vi "Init with Value.vi"(8 "error in":errorcluster, 10 "Value":variant, 11 "Check Box in":refnum<class "Check Box.lvclass">) -> (0 "error out":errorcluster, 3 "Check Box out":refnum<class "Check Box.lvclass">)   [LabVIEW 2024, in "SourceGrid.lvlib" / "Check Box.lvclass"]
uses:
  Check Box.lvclass
  Check Box.lvclass/Check Box.ctl
  Cells/Cell/Cell.lvclass
  D:/git/Sourcegrid-LabVIEW/source/Cells/Cell/Cell.lvclass
  D:/git/Sourcegrid-LabVIEW/source/Editors/Check Box/Check Box.lvclass
  D:/git/Sourcegrid-LabVIEW/dll/SourceGrid.dll
  dll/SourceGrid.dll
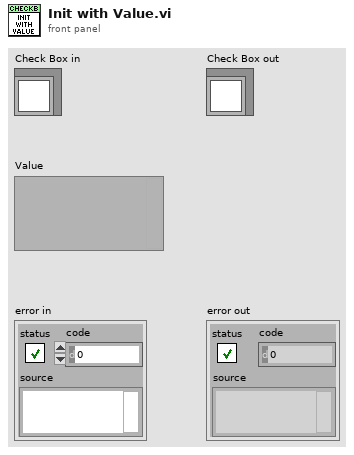
[diagram p1: front panel]
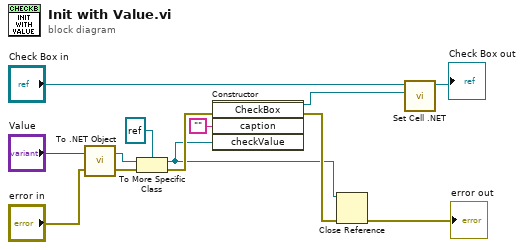
[diagram p0: block diagram]
diagram:
  n1 = call <vilib>:"To .NET Object.vi"("error in (no error)"="error in", "anything"="Value") -> ("error out"=w9:errorcluster, ".NET object"=w3:refnum<k24>)
  n2 = To More Specific Class(target class=refnum<k24> refnum ("checkValue"), reference=w3, error in=w9) -> (specific class reference=w2:refnum<k24>, error out=w8:errorcluster)
  n3 = constructor class="CheckBox"(error in=w8, "caption"="", "checkValue"=w2) -> (reference out=w1:refnum<k24>, error out=w13:errorcluster)  [unwired: 2 in, 3 out]
  n4 = Close Reference(reference=w2, error in (no error)=w13) -> (error out=→"error out":errorcluster)
  n5 = call "Set Cell .NET.vi"("Cell .NET"=w1, "Cell in"="Check Box in") -> ("Cell out"=→"Check Box out":refnum<class "Check Box.lvclass">)  [unwired: 9 in]
